vi "Reset Mutation History Helper.vi"() -> ()   [LabVIEW 2015, in "Utility.lvlib"]
uses:
  Utility.lvlib
panel:
  out "Mutations":i32[](array[numeric])
  out "After":i64 format="%.3p"
  out "Before":i64 format="%.3p"
  out "After":i64[](array[numeric])
  out "Before":i64[](array[numeric])
  out "file paths":path[](array[path])
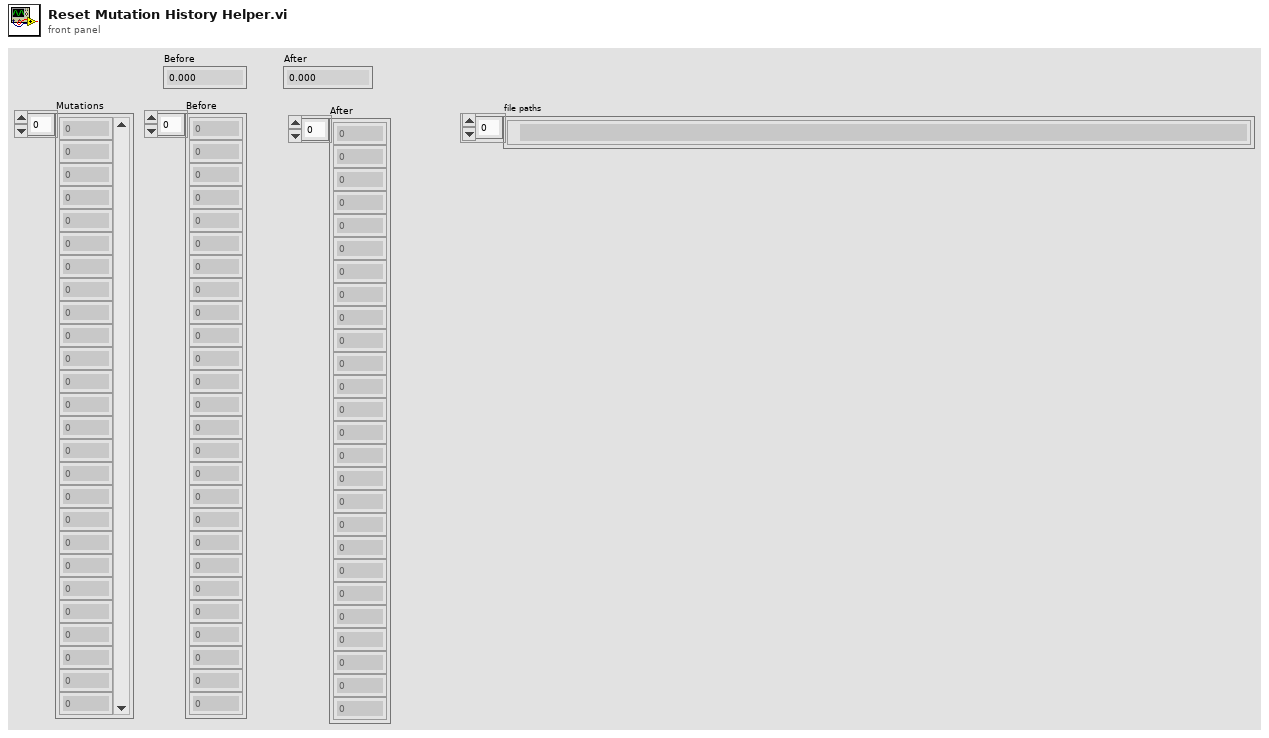
[diagram p1: front panel]
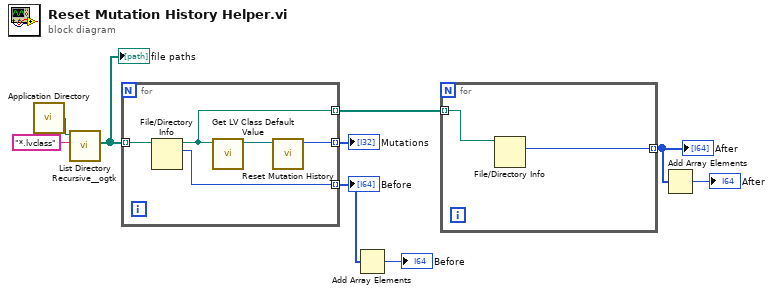
[diagram p0: block diagram]
diagram:
  n1 = call <vilib>:"Application Directory.vi"() -> ("Application Directory"=w7:path)
  n2 = call <userlib>:"List Directory Recursive__ogtk.vi"("pattern"="*.lvclass", "Path"=w7) -> ("file paths"=w8:path[])  [unwired: 6 in, 3 out]
  "file paths" <- w8
  n3 = for {
    tunnel: w8 -> [w14] mode=indexing
    tunnel: [w13] -> w5 mode=indexing
    tunnel: [w12] -> w6 mode=indexing
    tunnel: [w10] -> w1 mode=indexing
    n4 = File/Directory Info(path=w14) -> (path out=w12:path, size=w13:i64)  [unwired: 1 in, 5 out]
    n5 = call <vilib>:"Get LV Class Default Value.vi"("class path"=w12) -> ("object"=w11:refnum<class>)  [unwired: 9 in, 1 out]
    n6 = call "Reset Mutation History.vi"("LabVIEW Object"=w11) -> ("size(s)"=w10:i32)  [unwired: 10 in]
  }
  "Before" <- w5
  "Mutations" <- w1
  n7 = Add Array Elements(numeric array=w5) -> (sum=→"Before":i64)
  n8 = for {
    tunnel: w6 -> [w16] mode=indexing
    tunnel: [w15] -> w2 mode=indexing
    n9 = File/Directory Info(path=w16) -> (size=w15:i64)  [unwired: 1 in, 6 out]
  }
  "After" <- w2
  n10 = Add Array Elements(numeric array=w2) -> (sum=→"After":i64)
